vi "Check Accessors for Field.vi"(7 "Entity Path":path, 11 "Type":refnum<class "Type.lvclass">) -> (3 "Accessors":T1)   [LabVIEW 2020, in "Conditum-Tools.lvlib" / "Entity Editor.lvclass"]
uses:
  Entity Editor.lvclass
  <vilib>/IlluminatedG/IG Conditum Base/Conditum/Columns/Type/Type.lvclass
  Accessors.ctl
  Accessor Scope.ctl
  <vilib>/IlluminatedG/IG Conditum Base/Conditum/Columns/Type/Type.lvclass/Type.ctl
  <vilib>/xml/Load XML File.vi
  <vilib>/xml/Close Reference(Node).vi
  <vilib>/xml/NI_XML.lvlib
  Conditum-Tools.lvlib
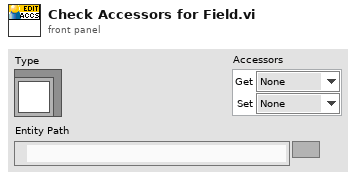
[diagram p1: front panel]
types:
  T1 = typedef "Conditum-Tools.lvlib/Accessors.ctl" = cluster{"Get":T2, "Set":T2}
  T2 = typedef "Conditum-Tools.lvlib/Accessor Scope.ctl" = enum16{"None", "Public", "Protected", "Private"}
  T3 = enum32{"invalid scope", "public", "private", "protected", "community"}
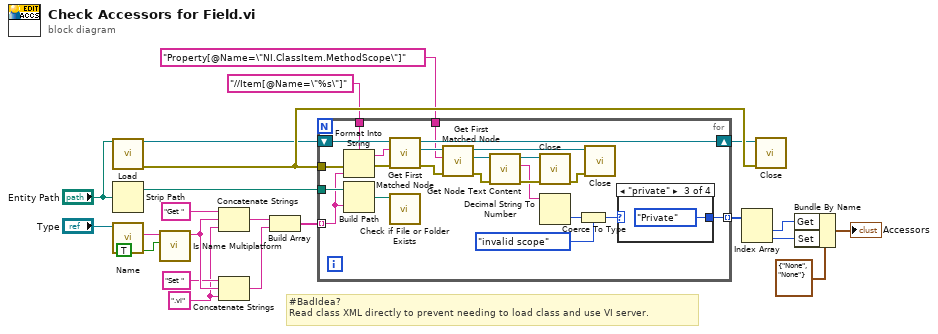
[diagram p0: block diagram]
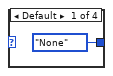
[diagram p2: hidden frame]
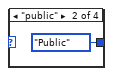
[diagram p3: hidden frame]
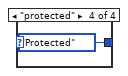
[diagram p4: hidden frame]
diagram:
  w16 = ".vi" ("string")
  # "#BadIdea?\nRead class XML directly to prevent needing to load class and use VI server."
  n1 = call-poly <vilib>:"Load.vi"("path to XML document"="Entity Path") -> ("DOM document out"=w14:refnum<k20>, "error out"=w22:errorcluster)  [unwired: 12 in, 1 out]
  n2 = Strip Path(path="Entity Path") -> (stripped path=w7:path)  [unwired: 1 out]
  n3 = call <vilib>:"Name.vi"("Type in"="Type") -> ("Table Name"=w1:string)  [unwired: 10 in]
  n4 = call <vilib>:"Is Name Multiplatform.vi"("filename must be valid on all platforms (F)"=TRUE, "filename"=w1) -> ("suggested filename"=w18:string)  [unwired: 5 in, 4 out]
  n5 = Concatenate Strings("Get " ("string"), w18, w16) -> (w10:string)
  n6 = Concatenate Strings("Set " ("string"), w18, w16) -> (w9:string)
  n7 = Build Array(w10, w9) -> (w8:string[])
  n8 = for {
    tunnel: "//Item[@Name=\"%s\"]" ("XPath expression") -> [w44]
    tunnel: w8 -> [w26] mode=indexing
    tunnel: "Property[@Name=\"NI.ClassItem.MethodScope\"]" ("XPath expression") -> [w30]
    shift-right: [w40] -> w12
    shift-left: w14 -> [w45]
    tunnel: w22 -> [w29]
    tunnel: w7 -> [w27]
    tunnel: [w23] -> w6 mode=indexing
    n9 = Format Into String(format string=w44, error in=w29, w26) -> (resulting string=w43:string, error out=w28:errorcluster)  [unwired: 1 in]
    n10 = Build Path(base path=w27, name or relative path=w26) -> (appended path=w25:path)
    n11 = call <vilib>:"Get First Matched Node.vi"("error in (no error)"=w28, "XPath expression"=w43, "node in"=w45) -> ("error out"=w36:errorcluster, "node result"=w41:refnum<k20>, "node out"=w40:refnum<k20>)  [unwired: 6 in]
    n12 = call <vilib>:"Check if File or Folder Exists.vi"("path"=w25) -> ()  [unwired: 8 in, 3 out]
    n13 = call <vilib>:"Get First Matched Node.vi"("error in (no error)"=w36, "XPath expression"=w30, "node in"=w41) -> ("error out"=w34:errorcluster, "node result"=w35:refnum<k20>, "node out"=w42:refnum<k20>)  [unwired: 6 in]
    n14 = call <vilib>:"Get Node Text Content.vi"("error in (no error)"=w34, "node in"=w35) -> ("error out"=w33:errorcluster, "node text"=w32:string, "node out"=w31:refnum<k20>)  [unwired: 7 in]
    n15 = call-poly <vilib>:"Close.vi"("error in (no error)"=w33, "node"=w31) -> ("error out"=w39:errorcluster)  [unwired: 7 in]
    n16 = Decimal String To Number(string=w32) -> (number=w38:i32)  [unwired: 2 in, 1 out]
    n17 = Coerce To Type(0:w38, 1:T3."invalid scope" ("Get Library Access Scope")) -> (2:w24:T3)
    n18 = call-poly <vilib>:"Close.vi"("error in (no error)"=w39, "node"=w42) -> ()  [unwired: 7 in, 1 out]
    n19 = case shown="\"private\"" w24 {
      tunnel: [Accessor_Scope."None" ("Get") Accessor_Scope."Public" ("Get") Accessor_Scope."Private" ("Get") Accessor_Scope."Protected" ("Get")] -> w23
      frame Default {
      }
      frame "public" {
      }
      frame "private" {
      }
      frame "protected" {
      }
    }
  }
  n20 = Index Array(array=w6) -> (element #1=w3:T2, element #2=w4:T2)  [unwired: 2 in]
  n21 = call-poly <vilib>:"Close.vi"("error in (no error)"=w22, "node"=w12) -> ()  [unwired: 7 in, 1 out]
  n22 = Bundle By Name(cluster=T1 {"Get"=enum."None", "Set"=enum."None"} ("Accessors"), "Get"=w3, "Set"=w4) -> (→"Accessors":T1)
